vi "Flatten Target Info To String.vi"(11 "Target Info":T1) -> (3 "Target Info String":string)   [LabVIEW 2014, in "LMH-LINX.lvlib"]
uses:
  <vilib>/MakerHub/LINX/LMH-LINX.lvlib
  <vilib>/MakerHub/LINX/Private/Utilties/Target Management/Target Info.ctl
  <vilib>/MakerHub/LINX/Private/Utilties/Target Management/NIC Info.ctl
  <vilib>/MakerHub/LINX/Private/Utilties/Target Management/NIC Mode.ctl
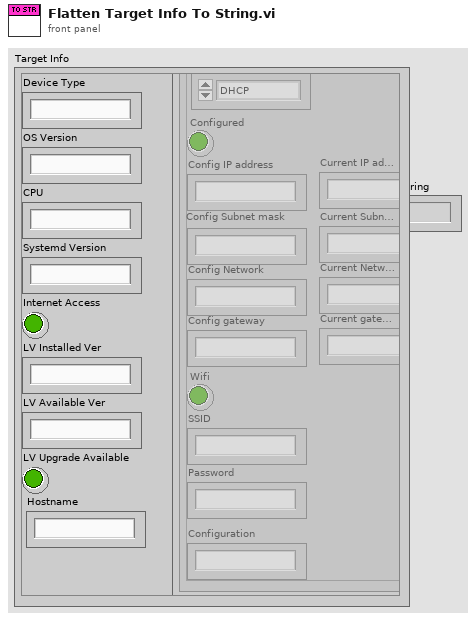
[diagram p1: front panel]
types:
  T1 = typedef "LMH-LINX.lvlib/Target Info.ctl" = cluster{"OS Version":string, "CPU":string, "Systemd Version":string, "Internet Access":bool, "Device Type":string, "LV Installed Ver":string, "LV Available Ver":string, "LV Upgrade Available":bool, "Hostname":string, "NIC Info":T2[]}
  T2 = typedef "LMH-LINX.lvlib/NIC Info.ctl" = cluster{"Name":string, "NIC Mode":T3, "Configured":bool, "Config IP address":string, "Config Subnet mask":string, "Config Network":string, "Config gateway":string, "Wifi":bool, "SSID":string, "Password":string, "Configuration":string, "Current IP address":string, "Current Subnet mask":string, "Current gateway":string, "Current Network":string}
  T3 = typedef "LMH-LINX.lvlib/NIC Mode.ctl" = enum16{"DHCP", "Static", "Loopback"}
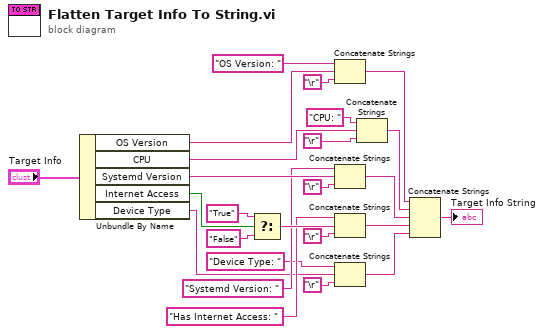
[diagram p0: block diagram]
diagram:
  n1 = Unbundle By Name("Target Info") -> ("OS Version"=w7:string, "CPU"=w12:string, "Systemd Version"=w13:string, "Internet Access"=w20:bool, "Device Type"=w3:string)
  n2 = Select(t="True", s=w20, f="False") -> (s? t:f=w17:string)
  n3 = Concatenate Strings("OS Version: ", w7, "\r") -> (w21:string)
  n4 = Concatenate Strings("Systemd Version: ", w13, "\r") -> (w23:string)
  n5 = Concatenate Strings("Has Internet Access: ", w17, "\r") -> (w24:string)
  n6 = Concatenate Strings("Device Type: " ("string"), w3, "\r") -> (w1:string)
  n7 = Concatenate Strings("CPU: ", w12, "\r") -> (w22:string)
  n8 = Concatenate Strings(w21, w22, w23, w24, w1) -> (→"Target Info String":string)
